vi "Configure Display Units.vi"(8 "error in (no error)":errorcluster, 9 "Units/Range (0: [A] Samples Per Second)":i32(ring) items=["[A] Samples Per Second", "[A] Hz", "[A] Seconds", "[P] Width Cycle", "[P] Duty Cycle", "[R] Hz", "[R] Seconds", "[S] Start Stop", "[S] Center Span", "[V] Amplitude Offset", "[V] High Low"], 10 "Type Operation (0: Arbitrary Waveform Rate Units)":i32(ring) items=["Arbitrary Waveform Rate Units", "Pulse Duration Units", "Rate Units", "Sweep Frequency Range", "Voltage Range"], 11 "VISA resource name":refnum<visa-resource-name>) -> (0 "error out":errorcluster, 3 "VISA resource name out":refnum<visa-resource-name>)   [LabVIEW 2023, in "Keysight-33500B.lvlib"]
doc: "Specifies the display units for arbitrary waveform, pulse duration, rate, sweep frequency range and voltage range.\n\n<b>Note</b>:\nThis VI is only applicable for 33611A, 33612A, 33621A and 33622A models."
uses:
  Keysight-33500B.lvlib
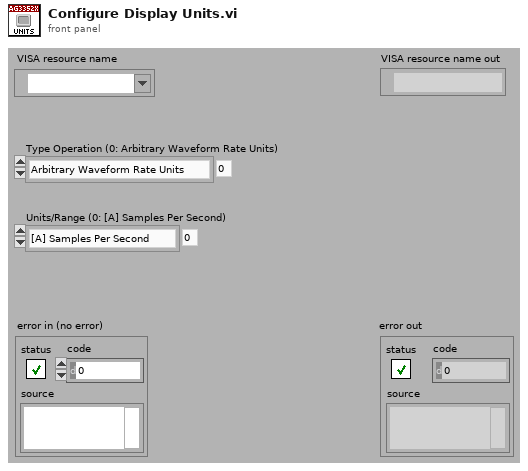
[diagram p1: front panel]
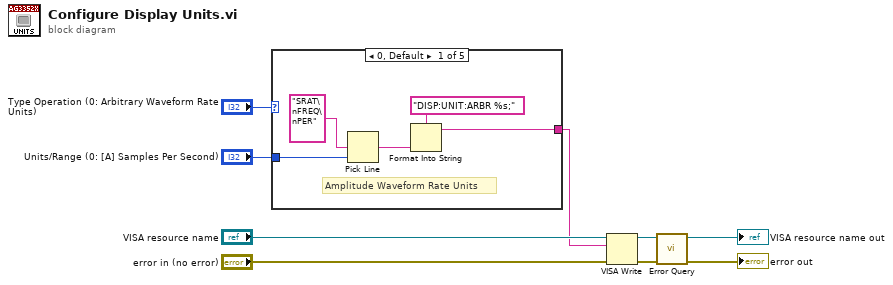
[diagram p0: block diagram]
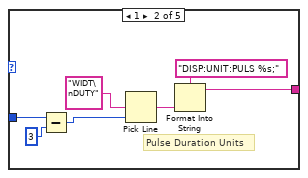
[diagram p2: hidden frame]
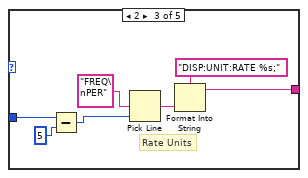
[diagram p3: hidden frame]
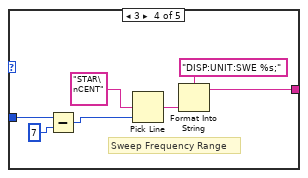
[diagram p4: hidden frame]
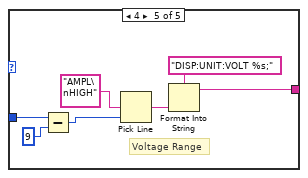
[diagram p5: hidden frame]
diagram:
  n1 = case shown="0, Default" "Type Operation (0: Arbitrary Waveform Rate Units)" {
    tunnel: "Units/Range (0: [A] Samples Per Second)" -> [w11 w17 w24 w31 w38]
    tunnel: [w10 w18 w25 w32 w39] -> w1
    frame 0, Default {
      # "Amplitude Waveform Rate Units"
      n2 = Pick Line(multi-line string="SRAT\nFREQ\nPER", line index=w11) -> (output string=w14:string)  [unwired: 1 out]
      n3 = Format Into String(format string="DISP:UNIT:ARBR %s;", w14) -> (resulting string=w10:string)  [unwired: 2 in, 1 out]
    }
    frame 1 {
      # "Pulse Duration Units"
      n4 = Subtract(x=w17, y=3) -> (x-y=w15:i32)
      n5 = Pick Line(multi-line string="WIDT\nDUTY", line index=w15) -> (output string=w21:string)  [unwired: 1 out]
      n6 = Format Into String(format string="DISP:UNIT:PULS %s;", w21) -> (resulting string=w18:string)  [unwired: 2 in, 1 out]
    }
    frame 2 {
      # "Rate Units"
      n7 = Subtract(x=w24, y=5) -> (x-y=w22:i32)
      n8 = Pick Line(multi-line string="FREQ\nPER", line index=w22) -> (output string=w28:string)  [unwired: 1 out]
      n9 = Format Into String(format string="DISP:UNIT:RATE %s;", w28) -> (resulting string=w25:string)  [unwired: 2 in, 1 out]
    }
    frame 3 {
      # "Sweep Frequency Range"
      n10 = Subtract(x=w31, y=7) -> (x-y=w29:i32)
      n11 = Pick Line(multi-line string="STAR\nCENT", line index=w29) -> (output string=w35:string)  [unwired: 1 out]
      n12 = Format Into String(format string="DISP:UNIT:SWE %s;", w35) -> (resulting string=w32:string)  [unwired: 2 in, 1 out]
    }
    frame 4 {
      # "Voltage Range"
      n13 = Subtract(x=w38, y=9) -> (x-y=w36:i32)
      n14 = Pick Line(multi-line string="AMPL\nHIGH", line index=w36) -> (output string=w42:string)  [unwired: 1 out]
      n15 = Format Into String(format string="DISP:UNIT:VOLT %s;", w42) -> (resulting string=w39:string)  [unwired: 2 in, 1 out]
    }
  }
  n16 = VISA Write(VISA resource name="VISA resource name", write buffer=w1, error in (no error)="error in (no error)") -> (VISA resource name out=w7:refnum<visa-resource-name>, error out=w6:errorcluster)  [unwired: 1 out]
  n17 = call "Error Query.vi"("error in (no error)"=w6, "VISA resource name"=w7) -> ("error out"=→"error out":errorcluster, "VISA resource name out"=→"VISA resource name out":refnum<visa-resource-name>)  [unwired: 8 out]
